vi "RVC Multi-dimensional Case.vi"() -> ()   [LabVIEW 2013]
panel:
  out "position 2":cluster{dbl[], "P(A)":dbl[]}[](graph)
  out "position":cluster{dbl[], "P(A)":dbl[]}[](graph)
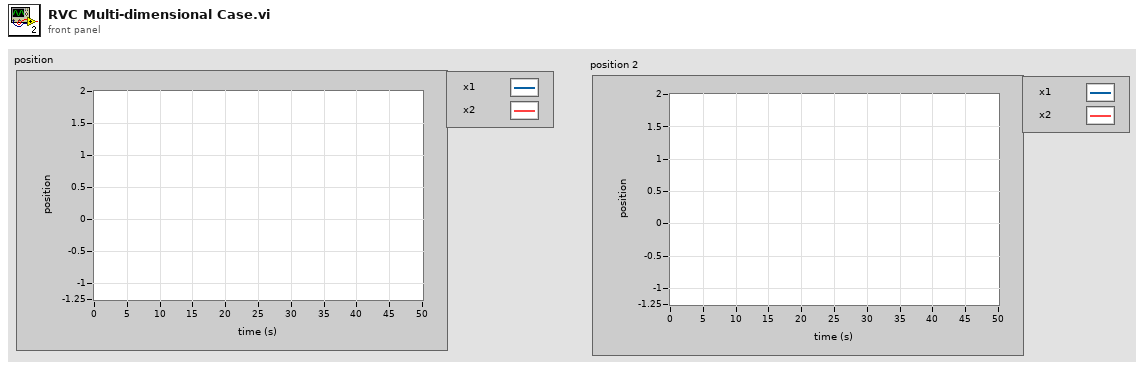
[diagram p1: front panel]
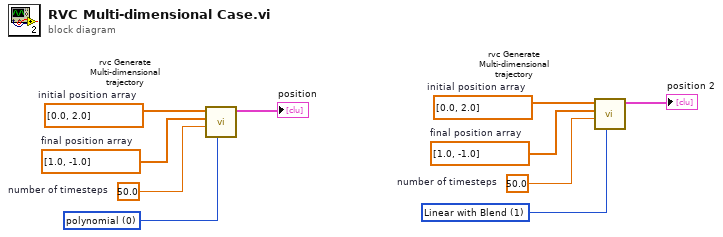
[diagram p0: block diagram]
diagram:
  w5 = u16 1 items=["polynomial", "Linear with Blend"] ("type of interpolator")
  w3 = 50.0  # number of timesteps
  w2 = dbl[] [1.0, -1.0]  # final position array
  w1 = dbl[] [0.0, 2.0]  # initial position array
  w6 = u16 0 items=["polynomial", "Linear with Blend"] ("type of interpolator")
  w8 = 50.0  # number of timesteps
  w9 = dbl[] [1.0, -1.0]  # final position array
  w10 = dbl[] [0.0, 2.0]  # initial position array
  n1 = call "rvc Generate Multi-dimensional trajectory.vi"("type of interpolator"=w6, "number of timesteps"=w8, "final position array"=w9, "initial position array"=w10) -> ("position"=→"position":cluster{dbl[], "P(A)":dbl[]}[])  [unwired: 4 in, 3 out]
  n2 = call "rvc Generate Multi-dimensional trajectory.vi"("type of interpolator"=w5, "number of timesteps"=w3, "final position array"=w2, "initial position array"=w1) -> ("position"=→"position 2":cluster{dbl[], "P(A)":dbl[]}[])  [unwired: 4 in, 3 out]
